vi "Friction Factor.vi"(10 "Effective Length":dbl, 11 "Reynolds Number":dbl) -> (3 "Friction Factor":dbl)   [LabVIEW 2019]
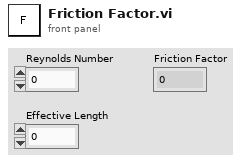
[diagram p1: front panel]
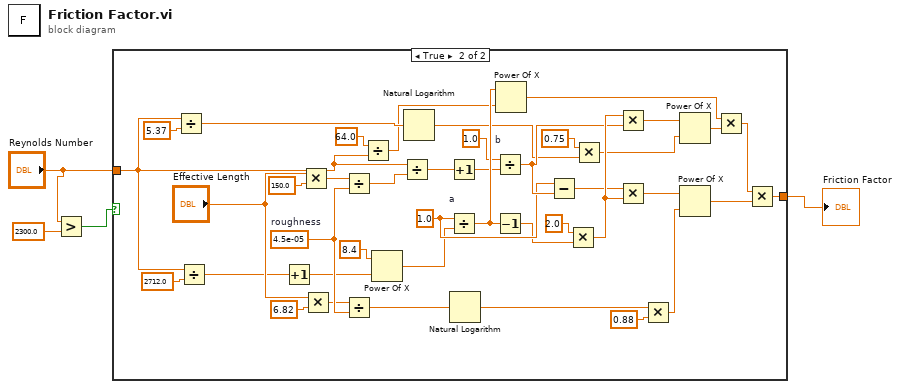
[diagram p0: block diagram]
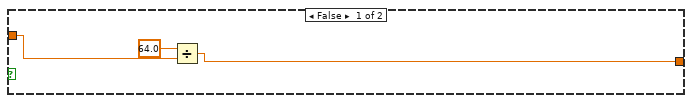
[diagram p2: hidden frame]
diagram:
  n1 = Greater?(x="Reynolds Number", y=2300.0) -> (0:w1:bool)
  n2 = case shown="True" w1 {
    tunnel: [w5 w48] -> w4
    tunnel: "Reynolds Number" -> [w7 w24]
    frame False {
      n3 = Divide(x=64.0, y=w7) -> (x/y=w5:dbl)
    }
    frame True {
      w38 = 4.5e-05  # roughness
      w42 = 1.0
      n4 = Divide(x=w24, y=5.37) -> (x/y=w25:dbl)
      n5 = Divide(x=w24, y=2712.0) -> (x/y=w9:dbl)
      n6 = Increment(x=w9) -> (x+1=w10:dbl)
      n7 = Multiply(x="Effective Length", y=150.0) -> (x*y=w16:dbl)
      n8 = Multiply(x="Effective Length", y=6.82) -> (x*y=w37:dbl)
      n9 = Divide(x=w16, y=w38) -> (x/y=w17:dbl)
      n10 = Divide(x=w37, y=w38) -> (x/y=w39:dbl)
      n11 = Divide(x=64.0, y=w24) -> (x/y=w20:dbl)
      n12 = Power Of X(1:w10, 2:8.4) -> (0:w12:dbl)
      n13 = Divide(x=w24, y=w17) -> (x/y=w14:dbl)
      n14 = Natural Logarithm(1:w25) -> (0:w26:dbl)
      n15 = Increment(x=w14) -> (x+1=w18:dbl)
      n16 = Divide "a"(x=w42, y=w12) -> (x/y=w29:dbl)
      n17 = Natural Logarithm(1:w39) -> (0:w40:dbl)
      n18 = Divide "b"(x=1.0, y=w18) -> (x/y=w43:dbl)
      n19 = Decrement(x=w29) -> (x-1=w30:dbl)
      n20 = Power Of X(1:w20, 2:w29) -> (0:w21:dbl)
      n21 = Subtract(x=w42, y=w43) -> (x-y=w44:dbl)
      n22 = Multiply(x=2.0, y=w30) -> (x*y=w45:dbl)
      n23 = Multiply(x=0.75, y=w26) -> (x*y=w27:dbl)
      n24 = Multiply(x=w45, y=w43) -> (x*y=w31:dbl)
      n25 = Multiply(x=w44, y=w45) -> (x*y=w46:dbl)
      n26 = Multiply(x=w40, y=0.88) -> (x*y=w41:dbl)
      n27 = Power Of X(1:w27, 2:w31) -> (0:w32:dbl)
      n28 = Power Of X(1:w41, 2:w46) -> (0:w47:dbl)
      n29 = Multiply(x=w21, y=w32) -> (x*y=w33:dbl)
      n30 = Multiply(x=w33, y=w47) -> (x*y=w48:dbl)
    }
  }
  "Friction Factor" <- w4
